vi "PH_OceanOpticsSpectrometer.panel.vi"(0 "object ref":refnum<vi>, 5 "error in (no error)":errorcluster) -> (19 "error out":errorcluster)   [LabVIEW 2014, in "PH_OceanOpticsSpectrometer.lvlib"]
doc: "By this VI a ross relais can be monitored and switched. \n\nThe indicators \"CLOSED\", \"OPEN\" and \"SWITCH STATE\" show the value of the Beckhoff-Tag: blue indicates bad tag status reference problems, darkgreen false and lightgreen on. If everything is working fine, \"CLOSED\" and \"SWITCH STATE\" should show the same value, while \"OPEN\" has the opposite value. \n\nThe oval button switches the ross relais. It should be in the same state as the \"SWITCH STATE\" indicator. \n\n\"EXIT\" closes the front panel (GUI), while \"Delete Instance\" disconnects and removes the instance from the PCS.\n\nThis VI has no machine safety relevant logic: there is neither a check of internal conclict nor with other objects, for example conflict with other ross relais. Therefore it must be handled with care and should be operated by well educated operators only. It is forseen exclusively for direct operating and testing of the system. \n\nLicense Agreement for this software:\n\nCopyright (C)\nGesellschaft für Schwerionenforschung, GSI\nPlanckstr. 1\n64291 Darmstadt\nGermany\n\nContact: D.Beck@gsi.de \n\nThis program is free software; you can redistribute it and/or modify it under the terms of the GNU General Public License as published by the Free Software Foundation; either version 2 of the license, or (at your option) any later version.\n\nThis program is distributed in the hope that it will be useful, but WITHOUT ANYW ARRANTY; without even the implied warranty of MERCHANTABILITY or FITNESS FOR A PARTICULAR PURPOSE. See the GNU General License for more details (http://www.gnu.org).\n\nGesellschaft für Schwerionenforschung, GSI\nPlanckstr. 1, 64291 Darmstadt, Germany\nFor all questions and ideas contact: M.Richter@gsi.de, H.Brand@gsi.de or D.Beck@gsi.de.\nLast update: 18-DEC-2002"
uses:
  PH_OceanOpticsSpectrometer.lvlib
  PH_OceanOpticsSpectrometer.Trigger.ctl
  PH_Basics/PH_StatusHandler/PH_StatusHandler.GUI element.ctl
  CS_Core/CSObj/CSObj.lvlib
  PH_Basics/PH_Common/PH_Common.lvlib
  CS_Core/CSSystem/CSSystemLib/CSSystemLib.lvlib
  PH_Basics/PH_Class/PH_Class.lvlib
  PH_Basics/PH_PSDBWriter/PH_PSDBWriter.lvlib
  PH_Basics/PH_StatusHandler/PH_StatusHandler.lvlib
panel:
  out "Firmware Revision":string
  out "Driver Revision":string
  out "Model":string
  out "VISA resource name":refnum<visa-resource-name>
  out "PSDB Status":u32(colorbox)=6618880 caption="PSDB"
  out "Trigger Info":string="Trigger Info"
  out "Status":T1
  out "Current Trigger Mode":T2=enum."Normal" caption="Current"
  out "center wavelength":sgl format="%#.1f"
  out "width":dbl format="%.1p"
  in  "Save":bool
  in  "Trigger Mode":T2=enum."Normal" caption="Wanted         Current"
  in  "Integration Time":u16=100 caption="ms"
  in  "Display Width":dbl(slide)=50.0 scale=10.0..200.0
  in  "Display Center":dbl(slide)=1054.0 scale=975.0..1125.0
  out "Spectrum":cluster{"Wavelength Bins":sgl[], sgl[]}(graph)
  in  "Delete":bool
  in  "Exit":bool
  # "PCS"
  # "3.40"
  # "+/-"
  # "nm"
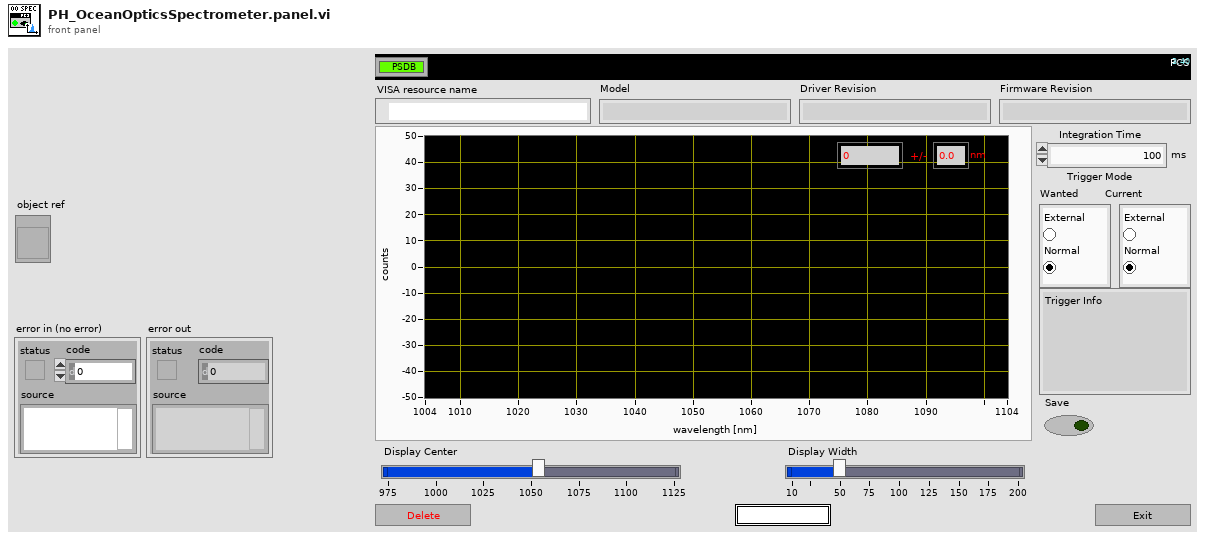
[diagram p1: front panel]
types:
  T1 = typedef "PH_StatusHandler.lvlib/PH_StatusHandler.GUI element.ctl" = u16
  T2 = typedef "PH_OceanOpticsSpectrometer.lvlib/PH_OceanOpticsSpectrometer.Trigger.ctl" = enum32{"External", "Normal"}
  T3 = typedef "PH_OceanOpticsSpectrometer.lvlib/PH_OceanOpticsSpectrometer.i attribute.ctl" = cluster{"GUI Refs":cluster{"Delete":refnum<vi>, "Spectrum":refnum<vi>, "Display Width":refnum<vi>, "Display Center":refnum<vi>, "Save":refnum<vi>, "Integration time":refnum<vi>, "center wavelength":refnum<vi>, "width":refnum<vi>, "Wanted Trigger Mode":refnum<vi>, "Current Trigger Mode":refnum<vi>, "Trigger Info":refnum<vi>, "Model":refnum<vi>, "Driver":refnum<vi>, "Firmware":refnum<vi>}, "Display":cluster{"Width":dbl, "Center":dbl}, "VISA resource name":refnum<visa-resource-name>, "Integration time [ms]":cluster{"Current Value":u16, "Wanted Value":u16}, "Trigger":cluster{"Current value":T2, "Wanted value":T2}, "Default VISA Timeout":u32, "Last Data":cluster{"Wavelength Bins":dbl[], "Spectrum by Pixels":dbl[]}}
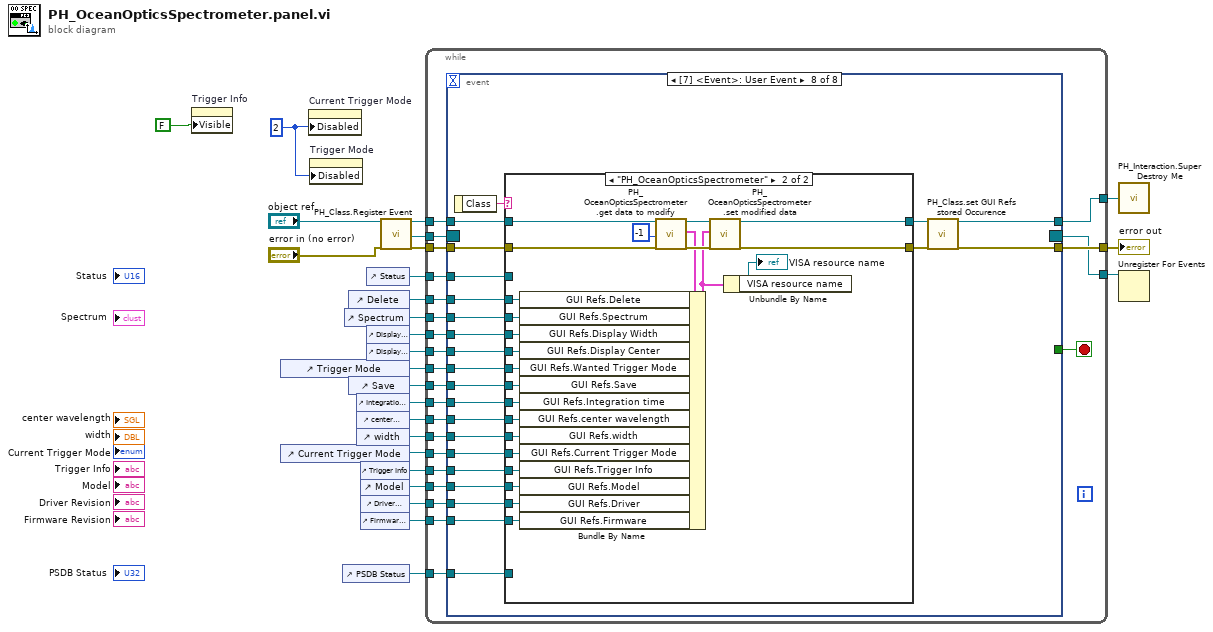
[diagram p0: block diagram]
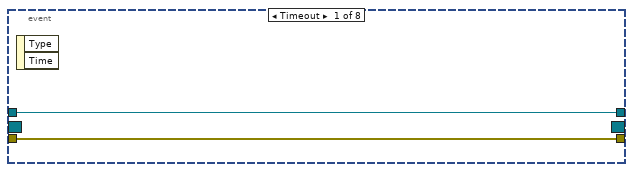
[diagram p2: hidden frame]
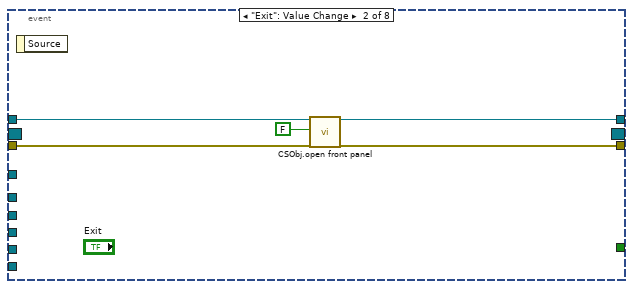
[diagram p3: hidden frame]
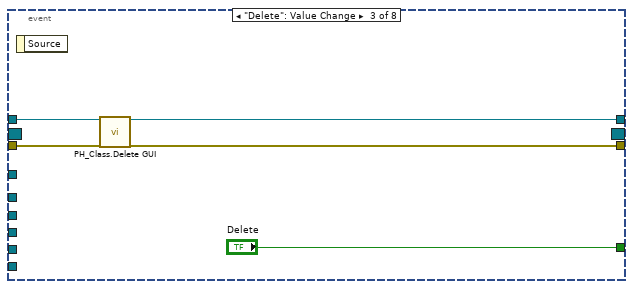
[diagram p4: hidden frame]
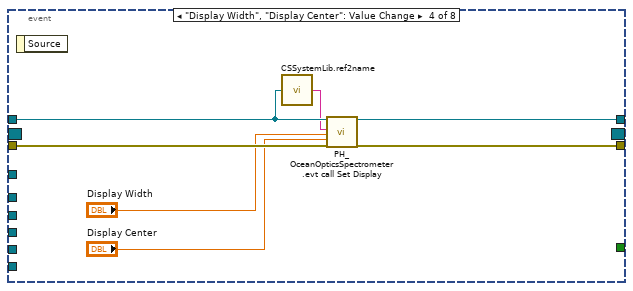
[diagram p5: hidden frame]
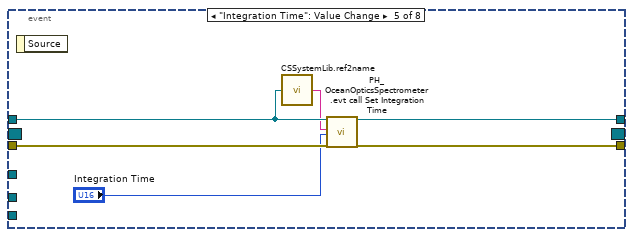
[diagram p6: hidden frame]
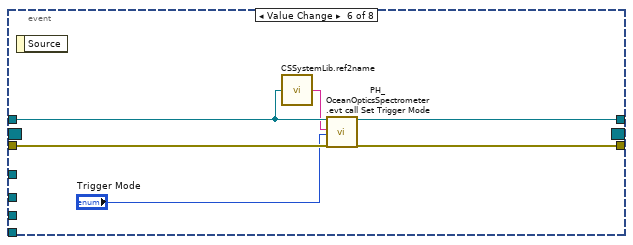
[diagram p7: hidden frame]
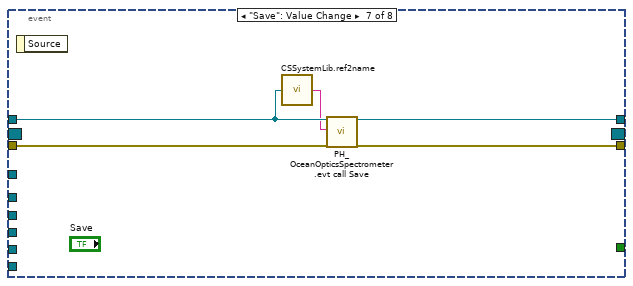
[diagram p8: hidden frame]
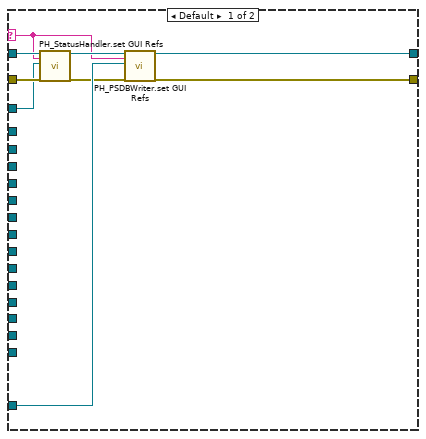
[diagram p9: hidden frame]
diagram:
  w24 = u8 2 ("Disabled")
  n1 = property on="Trigger Info" class="Str"("Visible"=FALSE) -> ()  [unwired: 2 in, 2 out]
  n2 = control-ref of="Trigger Mode"() -> (w11:refnum<vi>)
  n3 = control-ref of="Current Trigger Mode"() -> (w6:refnum<vi>)
  n4 = property on="Current Trigger Mode" class="RadioBtnsControl (strict)"("Disabled"=w24) -> ()  [unwired: 2 in, 2 out]
  n5 = property on="Trigger Mode" class="RadioBtnsControl (strict)"("Disabled"=w24) -> ()  [unwired: 2 in, 2 out]
  n6 = control-ref of="PSDB Status"() -> (w4:refnum<vi>)
  n7 = control-ref of="Spectrum"() -> (w14:refnum<vi>)
  n8 = control-ref of="Delete"() -> (w16:refnum<vi>)
  n9 = control-ref of="Save"() -> (w10:refnum<vi>)
  n10 = control-ref of="Integration Time"() -> (w9:refnum<vi>)
  n11 = control-ref of="center wavelength"() -> (w8:refnum<vi>)
  n12 = control-ref of="width"() -> (w7:refnum<vi>)
  n13 = control-ref of="Trigger Info"() -> (w5:refnum<vi>)
  n14 = control-ref of="Model"() -> (w3:refnum<vi>)
  n15 = control-ref of="Driver Revision"() -> (w2:refnum<vi>)
  n16 = control-ref of="Firmware Revision"() -> (w1:refnum<vi>)
  n17 = control-ref of="Status"() -> (w15:refnum<vi>)
  n18 = control-ref of="Display Width"() -> (w13:refnum<vi>)
  n19 = control-ref of="Display Center"() -> (w12:refnum<vi>)
  n20 = call "PH_Class.Register Event.vi"("i ref in"="object ref", "error in (no error)"="error in (no error)") -> ("i ref out"=w21:refnum<vi>, "Event Registration Refnum"=w20:refnum<event-registration>, "error out"=w22:errorcluster)  [unwired: 15 in]
  n21 = while {
    tunnel: w21 -> [w46]
    tunnel: [w45] -> w26
    tunnel: w22 -> [w48]
    tunnel: [w47] -> w25
    tunnel: w20 -> [w44]
    tunnel: [w43] -> w19
    tunnel: w16 -> [w42]
    tunnel: w15 -> [w41]
    tunnel: w14 -> [w40]
    tunnel: w13 -> [w39]
    tunnel: w12 -> [w38]
    tunnel: w11 -> [w37]
    tunnel: w10 -> [w36]
    tunnel: w9 -> [w35]
    tunnel: w8 -> [w34]
    tunnel: w7 -> [w33]
    tunnel: w6 -> [w32]
    tunnel: w5 -> [w31]
    tunnel: w4 -> [w30]
    tunnel: w3 -> [w29]
    tunnel: w2 -> [w28]
    tunnel: w1 -> [w27]
    stop <- w49 stop-if-true
    n22 = event shown="[7] <Event>: User Event" {
      selector: w44 -> [_ _ _ _ _ _ _ _]
      dyn-events: [_ _ _ _ _ _ _ _] -> w43
      timeout: _ -> [_ _ _ _ _ _ _ _]
      tunnel: [_ _ "Delete" _ _ _ _ _] -> w49
      tunnel: w46 -> [w50 w56 w59 w63 w71 w77 w82 w106]
      tunnel: w48 -> [w51 w54 w60 w68 w74 w80 w85 w105]
      tunnel: [w51 w53 w57 w66 w72 w78 w83 w107] -> w47
      tunnel: [w50 w52 w58 w67 w73 w79 w84 w108] -> w45
      tunnel: w42 -> [_ _ _ _ _ _ _ w101]
      tunnel: w41 -> [_ _ _ _ _ _ _ w100]
      tunnel: w40 -> [_ _ _ _ _ _ _ w99]
      tunnel: w39 -> [_ _ _ _ _ _ _ w98]
      tunnel: w38 -> [_ _ _ _ _ _ _ w97]
      tunnel: w37 -> [_ _ _ _ _ _ _ w96]
      tunnel: w36 -> [_ _ _ _ _ _ _ w95]
      tunnel: w35 -> [_ _ _ _ _ _ _ w94]
      tunnel: w34 -> [_ _ _ _ _ _ _ w93]
      tunnel: w33 -> [_ _ _ _ _ _ _ w92]
      tunnel: w32 -> [_ _ _ _ _ _ _ w91]
      tunnel: w31 -> [_ _ _ _ _ _ _ w90]
      tunnel: w30 -> [_ _ _ _ _ _ _ w89]
      tunnel: w29 -> [_ _ _ _ _ _ _ w88]
      tunnel: w28 -> [_ _ _ _ _ _ _ w87]
      tunnel: w27 -> [_ _ _ _ _ _ _ w86]
      event Timeout {
        n23 = event-data() -> ()  [unwired: 1 in, 2 out]
      }
      event "Exit": Value Change {
        n24 = event-data() -> ()  [unwired: 1 in, 1 out]
        n25 = call "CSObj.open front panel.vi"("i ref in"=w56, "frontPanelOpen"=FALSE ("front panel open"), "error in (no error)"=w54) -> ("i ref out"=w52:refnum<vi>, "error out"=w53:errorcluster)  [unwired: 15 in]
      }
      event "Delete": Value Change {
        n26 = event-data() -> ()  [unwired: 1 in, 1 out]
        n27 = call "PH_Class.Delete GUI.vi"("VI in"=w59, "error in (no error)"=w60) -> ("VI out"=w58:refnum<vi>, "error out"=w57:errorcluster)  [unwired: 16 in]
      }
      event "Display Width", "Display Center": Value Change {
        n28 = event-data() -> ()  [unwired: 1 in, 1 out]
        n29 = call "CSSystemLib.ref2name.vi"("obj refnum"=w63) -> ("name"=w62:string)
        n30 = call "PH_OceanOpticsSpectrometer.evt call Set Display.vi"("i ref in"=w63, "Instance"=w62, "Integration Time [ms]"="Display Width", "Center"="Display Center", "error in (no error)"=w68) -> ("i ref out"=w67:refnum<vi>, "error out"=w66:errorcluster)  [unwired: 13 in]
      }
      event "Integration Time": Value Change {
        n31 = event-data() -> ()  [unwired: 1 in, 1 out]
        n32 = call "CSSystemLib.ref2name.vi"("obj refnum"=w71) -> ("name"=w70:string)
        n33 = call "PH_OceanOpticsSpectrometer.evt call Set Integration Time.vi"("i ref in"=w71, "Instance"=w70, "Integration Time [ms]"="Integration Time", "error in (no error)"=w74) -> ("i ref out"=w73:refnum<vi>, "error out"=w72:errorcluster)  [unwired: 14 in]
      }
      event Value Change {
        n34 = event-data() -> ()  [unwired: 1 in, 1 out]
        n35 = call "CSSystemLib.ref2name.vi"("obj refnum"=w77) -> ("name"=w76:string)
        n36 = call "PH_OceanOpticsSpectrometer.evt call Set Trigger Mode.vi"("i ref in"=w77, "Instance"=w76, "Trigger Mode"="Trigger Mode", "error in (no error)"=w80) -> ("i ref out"=w79:refnum<vi>, "error out"=w78:errorcluster)  [unwired: 14 in]
      }
      event "Save": Value Change {
        n37 = event-data() -> ()  [unwired: 1 in, 1 out]
        n38 = call "CSSystemLib.ref2name.vi"("obj refnum"=w82) -> ("name"=w81:string)
        n39 = call "PH_OceanOpticsSpectrometer.evt call Save.vi"("i ref in"=w82, "Instance"=w81, "error in (no error)"=w85) -> ("i ref out"=w84:refnum<vi>, "error out"=w83:errorcluster)  [unwired: 15 in]
      }
      event User Event {
        n40 = event-data() -> ("Class"=w102:string)  [unwired: 1 in]
        n41 = case shown="\"PH_OceanOpticsSpectrometer\"" w102 {
          selector: w102 -> [w110 _]
          tunnel: w106 -> [w112 w137]
          tunnel: w105 -> [w116 w136]
          tunnel: [w115 w135] -> w104
          tunnel: [w117 w134] -> w103
          tunnel: w101 -> [_ w133]
          tunnel: w100 -> [w109 _]
          tunnel: w99 -> [_ w132]
          tunnel: w98 -> [_ w131]
          tunnel: w97 -> [_ w130]
          tunnel: w96 -> [_ w129]
          tunnel: w95 -> [_ w128]
          tunnel: w94 -> [_ w127]
          tunnel: w93 -> [_ w126]
          tunnel: w92 -> [_ w125]
          tunnel: w91 -> [_ w124]
          tunnel: w90 -> [_ w123]
          tunnel: w89 -> [w114 _]
          tunnel: w88 -> [_ w120]
          tunnel: w87 -> [_ w119]
          tunnel: w86 -> [_ w118]
          frame Default {
            n42 = call "PH_StatusHandler.set GUI Refs.vi"("i ref in"=w112, "Class"=w110, "GUI Ref"=w109, "error in (no error)"=w116) -> ("i ref out"=w111:refnum<vi>, "error out"=w113:errorcluster)  [unwired: 14 in]
            n43 = call "PH_PSDBWriter.set GUI Refs.vi"("i ref in"=w111, "Class"=w110, "Ref PSDB Status"=w114, "error in"=w113) -> ("i ref out"=w117:refnum<vi>, "error out"=w115:errorcluster)  [unwired: 14 in]
          }
          frame "PH_OceanOpticsSpectrometer" {
            n44 = call "PH_OceanOpticsSpectrometer.get data to modify.vi"("i ref in"=w137, "ms timeout (10000)"=-1, "error in (no error)"=w136) -> ("i ref out"=w141:refnum<vi>, "i attribute"=w139:T3, "error out"=w140:errorcluster)  [unwired: 13 in, 1 out]
            n45 = Bundle By Name(cluster=w139, "GUI Refs.Delete"=w133, "GUI Refs.Spectrum"=w132, "GUI Refs.Display Width"=w131, "GUI Refs.Display Center"=w130, "GUI Refs.Wanted Trigger Mode"=w129, "GUI Refs.Save"=w128, "GUI Refs.Integration time"=w127, "GUI Refs.center wavelength"=w126, "GUI Refs.width"=w125, "GUI Refs.Current Trigger Mode"=w124, "GUI Refs.Trigger Info"=w123, "GUI Refs.Model"=w120, "GUI Refs.Driver"=w119, "GUI Refs.Firmware"=w118) -> (w122:T3)
            n46 = call "PH_OceanOpticsSpectrometer.set modified data.vi"("i ref in"=w141, "i attribute"=w122, "error in (no error)"=w140) -> ("i ref out"=w134:refnum<vi>, "error out"=w135:errorcluster)  [unwired: 15 in]
            n47 = Unbundle By Name(w122) -> ("VISA resource name"=→"VISA resource name":refnum<visa-resource-name>)
          }
        }
        n48 = call "PH_Class.set GUI Refs stored Occurence.vi"("i ref in"=w103, "error in (no error)"=w104) -> ("i ref out"=w108:refnum<vi>, "error out"=w107:errorcluster)  [unwired: 16 in]
      }
    }
  }
  "error out" <- w25
  n49 = call "PH_Interaction.Super Destroy Me.vi"("i ref out"=w26) -> ()
  n50 = Unregister For Events(event registration refnum=w19) -> ()  [unwired: 1 in, 1 out]
